vi "start-stop-status_poller_backup.vi"() -> ()   [LabVIEW 2011]
uses:
  Pollers/ttm_poller_panel_class/ttmServer.lvclass
panel:
  in  "start":bool
  in  "stop":bool
  in  "status":bool
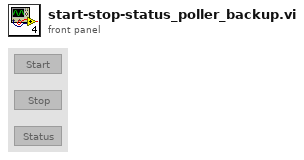
[diagram p1: front panel]
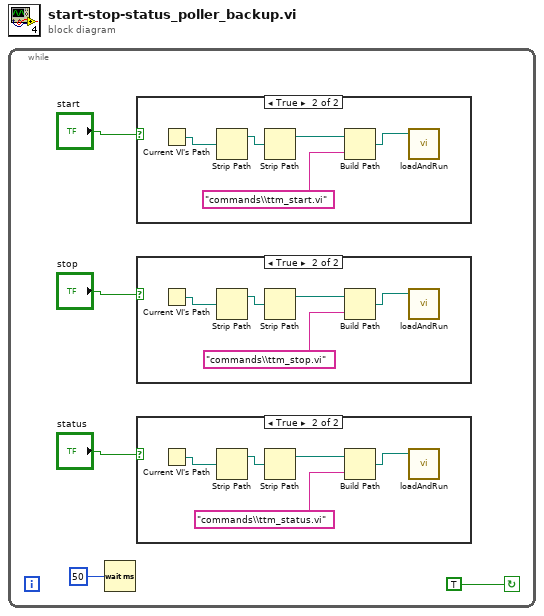
[diagram p0: block diagram]
diagram:
  n1 = while {
    stop <- TRUE continue-if-true
    n2 = Wait (ms)(milliseconds to wait=u32 50) -> ()  [unwired: 1 out]
    n3 = case shown="True" "start" {
      frame False {
      }
      frame True {
        n4 = Current VI's Path() -> (path=w20:path)
        n5 = Strip Path(path=w20) -> (stripped path=w19:path)  [unwired: 1 out]
        n6 = Strip Path(path=w19) -> (stripped path=w18:path)  [unwired: 1 out]
        n7 = Build Path(base path=w18, name or relative path="commands\\ttm_start.vi") -> (appended path=w16:path)
        n8 = call "loadAndRun.vi"("path"=w16) -> ()  [unwired: 3 in, 2 out]
      }
    }
    n9 = case shown="True" "stop" {
      frame False {
      }
      frame True {
        n10 = Current VI's Path() -> (path=w15:path)
        n11 = Strip Path(path=w15) -> (stripped path=w14:path)  [unwired: 1 out]
        n12 = Strip Path(path=w14) -> (stripped path=w13:path)  [unwired: 1 out]
        n13 = Build Path(base path=w13, name or relative path="commands\\ttm_stop.vi") -> (appended path=w11:path)
        n14 = call "loadAndRun.vi"("path"=w11) -> ()  [unwired: 3 in, 2 out]
      }
    }
    n15 = case shown="True" "status" {
      frame False {
      }
      frame True {
        n16 = Current VI's Path() -> (path=w10:path)
        n17 = Strip Path(path=w10) -> (stripped path=w9:path)  [unwired: 1 out]
        n18 = Strip Path(path=w9) -> (stripped path=w8:path)  [unwired: 1 out]
        n19 = Build Path(base path=w8, name or relative path="commands\\ttm_status.vi") -> (appended path=w6:path)
        n20 = call "loadAndRun.vi"("path"=w6) -> ()  [unwired: 3 in, 2 out]
      }
    }
  }
